vi "Calculate Sample Multiplier.vi"(0 "in DFE mode?":bool, 5 "prescale":u8, 7 "rx internal data width":T1=enum."32 Bit", 11 "error in":errorcluster) -> (4 "BER floor":dbl, 6 "sample multiplier":u64 max=63 format="%0d", 15 "error out":errorcluster)   [LabVIEW 2015, in "niHighSpeedSerial Eye Scan Common v1 Host.lvlib"]
doc: "Returns the sample multiplier, which is used to calculate the actual sample count from the unscaled sample count returned from the FPGA.\n\n<B>Input Parameters</B>\n\n<B>private data</B> is the class private data input into the VI.\n\n<B>private data.GTX2_CHANNEL register map</B> is the GTX2 Channel register map to use.\n\n<B>private data.instruction target</B> is the instruction target to use when communicating with the FPGA.\n\n<B>private data.channel measure state</B> maintains the internal state of the Eye Scan Single Point class.\nenum values: Uninitialized,Initialized,Ready,Request,Wait,Read,Process,Finished\n\n<B>private data.in DFE mode?</B> is true if Eye Scan is configured for DFE Equalization Mode.\n\n<B>private data.prescale</B> controls scaling of the sample count in order to keep the sample count and error count within reasonable precision.\n\n<B>private data.receiver data width</B> is the data width (in bits) of the receiver lane.\nenum values: 16 Bit,20 Bit,32 Bit,40 Bit\n\n<B>private data.active point</B> is the point currently being sampled for errors using Eye Scan.\n\n<B>private data.active point.horizontal offset</B> is the horizontal offset of the active point.\n\n<B>private data.active point.vertical offset</B> is the vertical offset of the active point.\n\n<B>private data.ut sign</B> The untapped threshold sign (positive or negative) currently configured on the point being measured.\nPositive is used when in DFE or LPM Equalization Mode, while Negative is only used in DFE Equalization Mode.\n\n<B>private data.positive counts</B> contains the number of sample and error counts measured using the positive UT Sign.\n\n<B>private data.positive counts.sample count</B> is the positive sample count when using DFE mode, or the entire sample count when using LPM mode.\n\n<B>private data.positive counts.error count</B> is the positive error count when using DFE mode, or the entire error count when using LPM mode.\n\n<B>private data.negative counts</B> contains the number of sample and error counts measured using the negative UT Sign.\n\n<B>private data.negative counts.sample count</B> is the negative sample count when using DFE mode, or unused when using LPM mode.\n\n<B>private data.negative counts.error count</B> is the negative error count when using DFE mode, or unused when using LPM mode.\n\n<B>error in</B> describes error conditions that occur before this node runs. This input provides standard 'error in' functionality.\n\n<B>Output Parameters</B>\n\n<B>private data out</B> is the class private data output from the VI.\n\n<B>private data out.GTX2_CHANNEL register map</B> is the register map to use which represents the GTX2 Channel.\n\n<B>private data out.instruction target</B> is the instruction target to use when communicating with the FPGA.\n\n<B>private data out.channel measure state</B> maintains the internal state of the Eye Scan Single Point class.\nenum values: Uninitialized,Initialized,Ready,Request,Wait,Read,Process,Finished\n\n<B>private data out.in DFE mode?</B> is true if Eye Scan is configured for DFE Equalization Mode.\n\n<B>private data out.prescale</B> controls scaling of the sample count in order to keep the sample count and error count within reasonable precision.\n\n<B>private data out.receiver data width</B> is the data width (in bits) of the receiver lane.\nenum values: 16 Bit,20 Bit,32 Bit,40 Bit\n\n<B>private data out.active point</B> is the point currently being sampled for errors using Eye Scan.\n\n<B>private data out.active point.horizontal offset</B> is the horizontal offset of the active point.\n\n<B>private data out.active point.vertical offset</B> is the vertical offset of the active point.\n\n<B>private data out.ut sign</B> contains the number of sample and error counts measured using the positive UT Sign.\nenum values: Positive,Negative\n\n<B>private data out.positive counts</B> contains the number of sample and error counts measured using the positive UT Sign.\n\n<B>private data out.positive counts.sample count</B> is the positive sample count when using DFE mode, or the entire sample count when using LPM mode.\n\n<B>private data out.positive counts.error count</B> is the positive error count when using DFE mode, or the entire error count when using LPM mode.\n\n<B>private data out.negative counts</B> contains the number of sample and error counts measured using the negative UT Sign.\n\n<B>private data out.negative counts.sample count</B> is the negative sample count when using DFE mode, or the entire sample count when using LPM mode.\n\n<B>private data out.negative counts.error count</B> is the negative error count when using DFE mode, or the entire error count when using LPM mode.\n\n<B>sample multiplier</B> is the value by which to multiply the unscaled sample count returned from the hardware to obtain the actual sample count.\n\n<B>error out</B> contains error information. This output provides standard 'error out' functionality."
uses:
  <instrlib>/niHighSpeedSerial/Eye Scan/v1/Host/Common/niHighSpeedSerial Eye Scan Common v1 Host.lvlib
  <instrlib>/niHighSpeedSerial/Eye Scan/v1/Host/Common/Public/Data Width.ctl
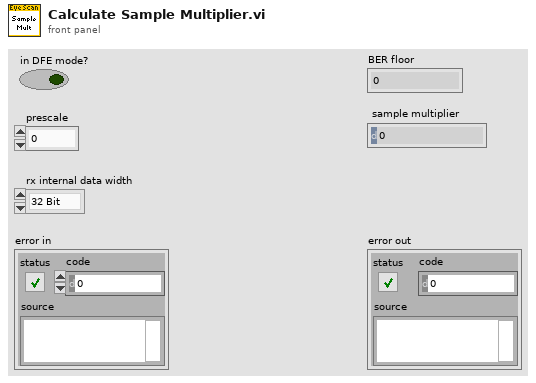
[diagram p1: front panel]
types:
  T1 = typedef "niHighSpeedSerial Eye Scan Common v1 Host.lvlib/Data Width.ctl" = enum16{"16 Bit", "20 Bit", "32 Bit", "40 Bit"}
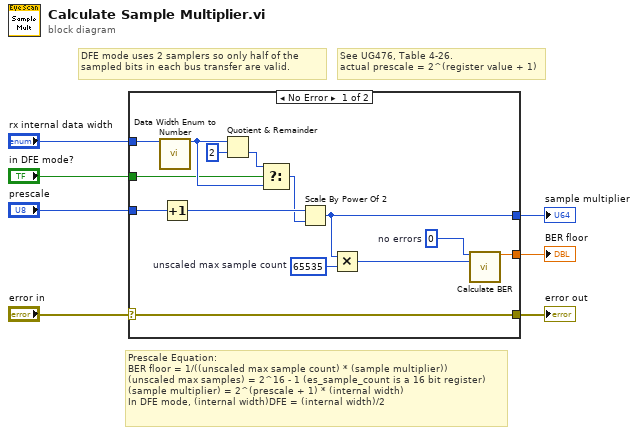
[diagram p0: block diagram]
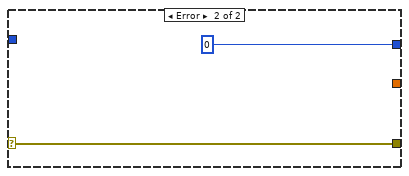
[diagram p2: hidden frame]
diagram:
  # "Prescale Equation:\nBER floor = 1/((unscaled max sample count) * (sample multiplier))\n(unscaled max samples) = 2^16 - 1 (es_sample_count is a 16 bit register)\n(sample multiplier) = 2^(prescale + 1) * (internal width)\nIn DFE mode, (internal width)DFE = (internal width)/2"
  # "DFE mode uses 2 samplers so only half of the sampled bits in each bus transfer are valid."
  # "See UG476, Table 4-26.\nactual prescale = 2^(register value + 1)"
  n1 = case shown="No Error" "error in" {
    selector: "error in" -> [w20 w23]
    tunnel: [w20 w23] -> w6
    tunnel: [w14 u64 0] -> w5
    tunnel: [w13 _] -> w4
    tunnel: "rx internal data width" -> [w10 _]
    tunnel: "in DFE mode?" -> [w9 _]
    tunnel: "prescale" -> [w8 _]
    frame No Error {
      w15 = u64 65535  # unscaled max sample count
      w11 = u64 0  # no errors
      n2 = call <instrlib>:"Data Width Enum to Number.vi"("receiver data width"=w10) -> ("numberic width"=w19:u64)  [unwired: 14 in]
      n3 = Increment(x=w8) -> (x+1=w21:u8)
      n4 = Quotient & Remainder(x=w19, y=u64 2) -> (floor(x/y)=w17:u64)  [unwired: 1 out]
      n5 = Select(t=w17, s=w9, f=w19) -> (s? t:f=w16:u64)
      n6 = Scale By Power Of 2(n=w21, x=w16) -> (x*2^n=w14:u64)
      n7 = Multiply(x=w14, y=w15) -> (x*y=w12:u64)
      n8 = call <instrlib>:"Calculate BER.vi"("error count"=w11, "sample count"=w12) -> ("BER"=w13:dbl)  [unwired: 13 in]
    }
    frame Error {
    }
  }
  "error out" <- w6
  "sample multiplier" <- w5
  "BER floor" <- w4
